vi "Prune below.vi"(1 "lower limit":dbl, 2 "Array in":dbl[](array[numeric])) -> (0 "Index out":i32)   [LabVIEW 2014]
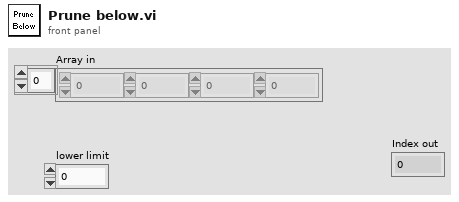
[diagram p1: front panel]
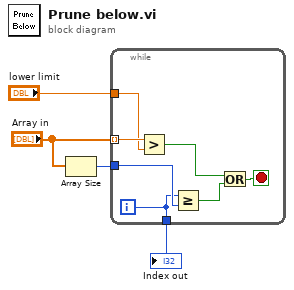
[diagram p0: block diagram]
diagram:
  n1 = Array Size(array="Array in") -> (size(s)=w3:i32)
  n2 = while {
    tunnel: "Array in" -> [w11] mode=indexing
    tunnel: w3 -> [w6]
    tunnel: "lower limit" -> [w10]
    tunnel: [w5] -> w1
    i -> [w5]
    stop <- w9 stop-if-true
    n3 = Greater?(x=w11, y=w10) -> (0:w8:bool)
    n4 = Greater Or Equal?(x=w5, y=w6) -> (x >= y?=w7:bool)
    n5 = Or(x=w8, y=w7) -> (x .or. y?=w9:bool)
  }
  "Index out" <- w1
